vi "CorSetAmplitude.vi"(8 "error in (no error)":errorcluster, 10 "Electrode Amplitudes":sgl[](array[numeric]), 11 "Cohort in":refnum<class "Cohort.lvclass">) -> (0 "error out":errorcluster, 3 "Cohort out":refnum<class "Cohort.lvclass">)   [LabVIEW 2012, in "Cohort.lvclass"]
uses:
  Cohort.lvclass
  Cohort.lvclass/Cohort.ctl
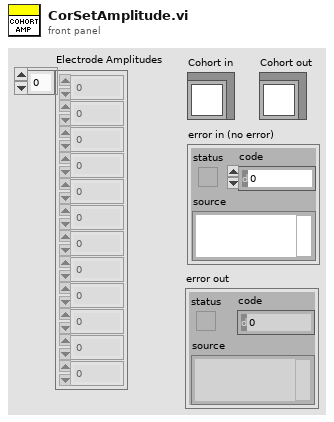
[diagram p1: front panel]
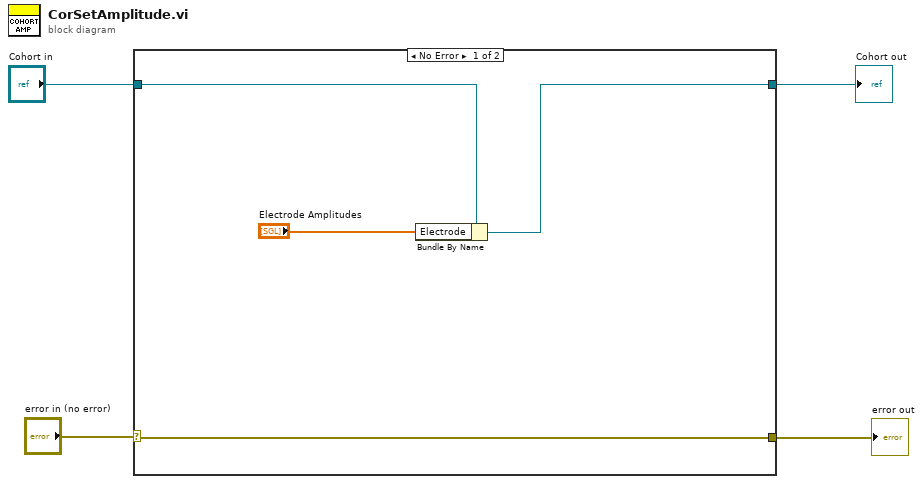
[diagram p0: block diagram]
diagram:
  n1 = case shown="No Error" "error in (no error)" {
    selector: "error in (no error)" -> [w6 w9]
    tunnel: [w6 w9] -> w3
    tunnel: [w8 w10] -> w1
    tunnel: "Cohort in" -> [w7 w10]
    frame No Error {
      n2 = Bundle By Name(cluster=w7, "Electrode"="Electrode Amplitudes") -> (w8:refnum<class "Cohort.lvclass">)
    }
    frame Error {
    }
  }
  "error out" <- w3
  "Cohort out" <- w1
